vi "Construct.vi"(8 "error in":errorcluster, 10 "Variant":variant, 11 "SUB in":refnum<class "SUB.lvclass">) -> (0 "error out":errorcluster, 3 "SUB out":refnum<class "SUB.lvclass">)   [LabVIEW 2014, in "SUB.lvclass"]
uses:
  SUB.lvclass
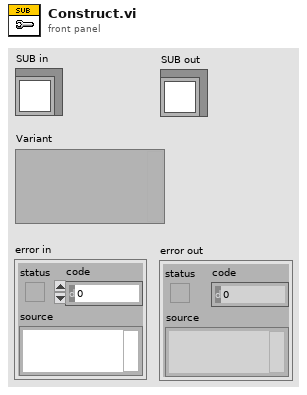
[diagram p1: front panel]
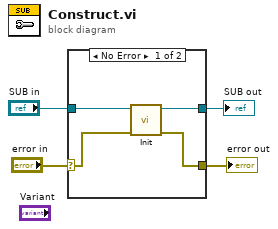
[diagram p0: block diagram]
diagram:
  n1 = case shown="No Error" "error in" {
    selector: "error in" -> [w6 w10]
    tunnel: [w7 w10] -> w3
    tunnel: [w8 w9] -> w1
    tunnel: "SUB in" -> [w5 w9]
    frame No Error {
      n2 = call-dynamic "Init.vi"("error in"=w6, "SEQ in"=w5) -> ("error out"=w7:errorcluster, "SEQ out"=w8:refnum<class "SUB.lvclass">)  [unwired: 8 in]
    }
    frame Error {
    }
  }
  "error out" <- w3
  "SUB out" <- w1
